vi "Array_Remove duplicates.vi"(8 "error in (no error)":errorcluster, 10 "Array Input":T1) -> (0 "error out":errorcluster, 2 "Array Output":T1)   [LabVIEW 2016, in "pickering.lvclass"]
uses:
  pickering.lvclass
  Typedefs/Channels-Array.ctl
  Typedefs/Channel-Cluster.ctl
  Typedefs/ChannelX-ComboBox.ctl
  Typedefs/ChannelY-ComboBox.ctl
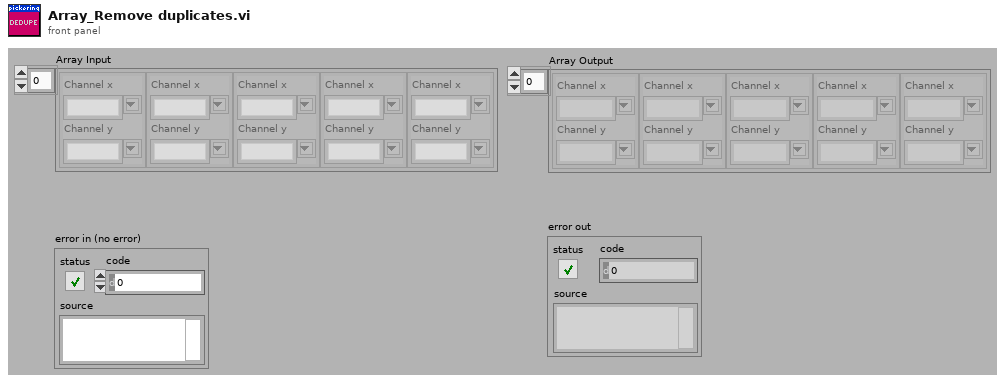
[diagram p1: front panel]
types:
  T1 = typedef "pickering.lvclass/Channels-Array.ctl" = T2[]
  T2 = typedef "pickering.lvclass/Channel-Cluster.ctl" = cluster{"Channel x":T3, "Channel y":T4}
  T3 = typedef "pickering.lvclass/ChannelX-ComboBox.ctl" = string
  T4 = typedef "pickering.lvclass/ChannelY-ComboBox.ctl" = string
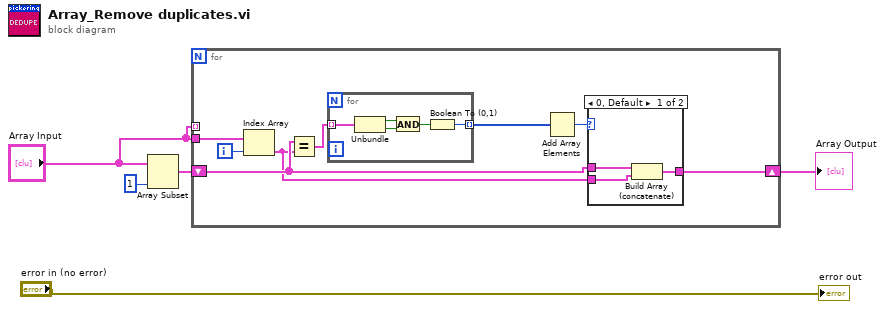
[diagram p0: block diagram]
diagram:
  n1 = Array Subset(array="Array Input", length=1) -> (w4:T1)  [unwired: 1 in]
  n2 = for {
    tunnel: "Array Input" -> [w13]
    shift-right: [w8] -> w2
    shift-left: w4 -> [w10]
    tunnel: "Array Input" -> [_] mode=indexing
    i -> [w12]
    n3 = Index Array(array=w13, index=w12) -> (element=w9:T2)
    n4 = Equal?(x=w10, y=w9) -> (x = y?=w7:cluster{"Channel x":bool, "Channel y":bool}[])
    n5 = for {
      tunnel: w7 -> [w22] mode=indexing
      tunnel: [w18] -> w6 mode=indexing
      n6 = Unbundle(w22) -> ("Channel x"=w21:bool, "Channel y"=w20:bool)
      n7 = And(x=w21, y=w20) -> (x .and. y?=w19:bool)
      n8 = Boolean To (0,1)(Boolean=w19) -> (0, 1=w18:i16)
    }
    n9 = Add Array Elements(numeric array=w6) -> (sum=w11:i16)
    n10 = case shown="0, Default" w11 {
      tunnel: w10 -> [w16 w17]
      tunnel: w9 -> [w15 _]
      tunnel: [w14 w17] -> w8
      frame 0, Default {
        n11 = Build Array (concatenate)(w16, w15) -> (w14:T1)
      }
      frame 1 {
      }
    }
  }
  "Array Output" <- w2
  "error out" <- "error in (no error)"
